vi "Strafe Rotate Math.vi"(8 "Theta Turn":dbl, 9 "Theta Forward":dbl, 10 "Turn Speed":dbl, 11 "Forward Speed":dbl) -> (2 "Target Rotation":dbl)   [LabVIEW 2020]
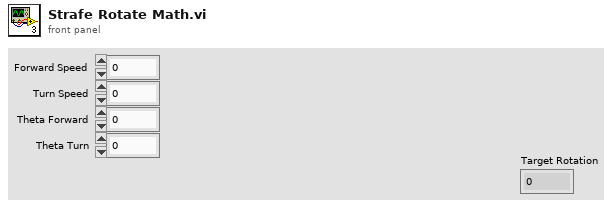
[diagram p1: front panel]
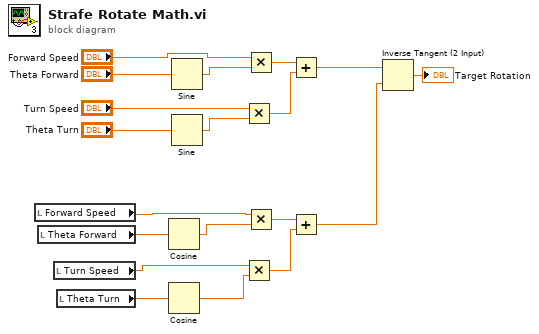
[diagram p0: block diagram]
diagram:
  n1 = local read "Forward Speed"() -> (w8:dbl)
  n2 = local read "Theta Forward"() -> (w11:dbl)
  n3 = local read "Turn Speed"() -> (w4:dbl)
  n4 = local read "Theta Turn"() -> (w6:dbl)
  n5 = Cosine(x=w11) -> (cos(x)=w7:dbl)
  n6 = Cosine(x=w6) -> (cos(x)=w5:dbl)
  n7 = Sine(x="Theta Forward") -> (sin(x)=w17:dbl)
  n8 = Sine(x="Theta Turn") -> (sin(x)=w13:dbl)
  n9 = Multiply(x="Turn Speed", y=w13) -> (x*y=w12:dbl)
  n10 = Multiply(x=w4, y=w5) -> (x*y=w10:dbl)
  n11 = Multiply(x="Forward Speed", y=w17) -> (x*y=w16:dbl)
  n12 = Multiply(x=w8, y=w7) -> (x*y=w9:dbl)
  n13 = Add(x=w16, y=w12) -> (x+y=w3:dbl)
  n14 = Add(x=w9, y=w10) -> (x+y=w2:dbl)
  n15 = Inverse Tangent (2 Input)(1:w2, 2:w3) -> (0:→"Target Rotation":dbl)
